vi "get_enabled_state.vi"(8 "error in (no error)":errorcluster, 11 "GenericClock in":refnum<class "GenericClock.lvclass">) -> (0 "error out":errorcluster, 2 "enabled?":bool, 3 "GenericClock out":refnum<class "GenericClock.lvclass">)   [LabVIEW 2017, in "GenericClock.lvclass"]
uses:
  GenericClock.lvclass
  GenericClock.lvclass/GenericClock.ctl
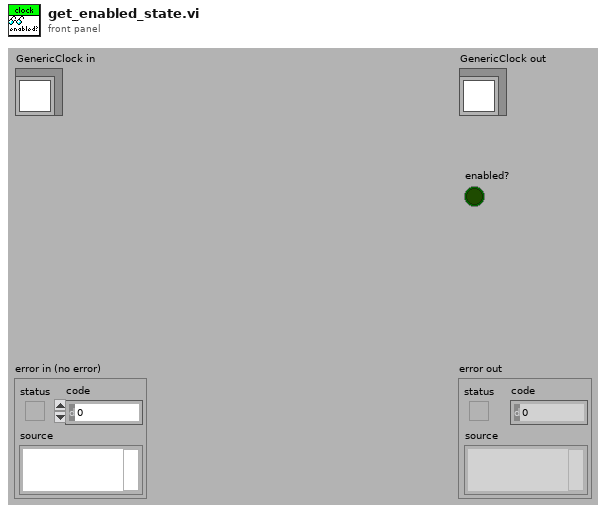
[diagram p1: front panel]
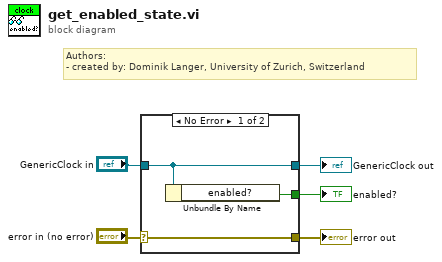
[diagram p0: block diagram]
diagram:
  # "Authors: \n- created by: Dominik Langer, University of Zurich, Switzerland"
  n1 = case shown="No Error" "error in (no error)" {
    selector: "error in (no error)" -> [w8 w10]
    tunnel: [w8 w10] -> w4
    tunnel: [w7 w9] -> w2
    tunnel: "GenericClock in" -> [w7 w9]
    tunnel: [w6 _] -> w1
    frame No Error {
      n2 = Unbundle By Name(w7) -> ("enabled?"=w6:bool)
    }
    frame Error {
    }
  }
  "error out" <- w4
  "GenericClock out" <- w2
  "enabled?" <- w1
